vi "Set BG Image.vi"(8 "error in (no error)":errorcluster, 11 "IMAQ Display in":refnum<class "HIJ IMAQdx Display.lvclass">) -> (0 "error out":errorcluster, 3 "IMAQ Display out":refnum<class "HIJ IMAQdx Display.lvclass">)   [LabVIEW 2020, in "HIJ IMAQdx Display.lvlib" / "HIJ IMAQdx Display.lvclass"]
uses:
  HIJ IMAQdx Display.lvclass
  C:/POLARIS Programme/POLARIS-AS-3-Cams/Submodules/HIJ Vision/Display Actors/HIJ Vision Display/HIJ Vision Display/HIJ Vision Display.lvclass
  HIJ IMAQdx Display.lvclass/HIJ IMAQdx Display.ctl
  HIJ Vision Display/HIJ Vision Display/HIJ Vision Display.lvclass/HIJ Vision Display.ctl
  HIJ Vision Display/HIJ Vision Display/Read Image Source Name.vi
  HIJ Vision Display/HIJ Vision Display/Read Display Image.vi
  HIJ Vision Display/HIJ Vision Display/Write Image Name Prefix.vi
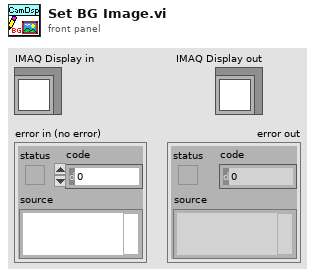
[diagram p1: front panel]
types:
  T1 = typedef "IMAQ Image.ctl" = refnum<image>
  T2 = typedef "Image Type" = u32
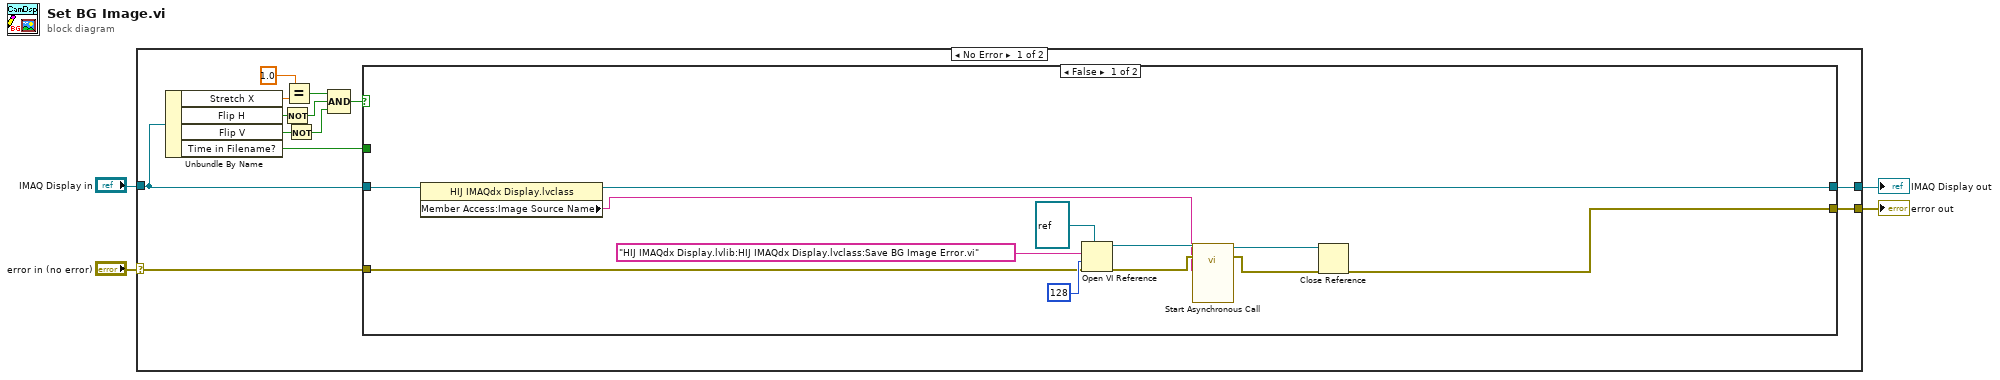
[diagram p0: block diagram]
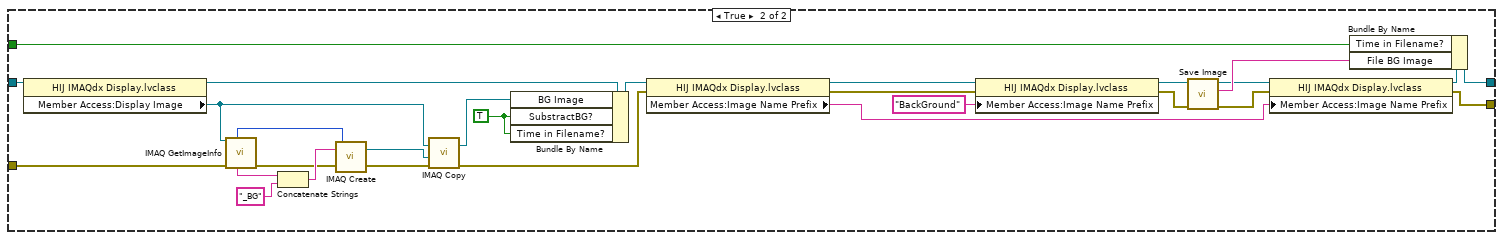
[diagram p2: hidden frame]
diagram:
  n1 = case shown="No Error" "error in (no error)" {
    selector: "error in (no error)" -> [w17 w58]
    tunnel: [w14 w58] -> w3
    tunnel: [w16 w59] -> w1
    tunnel: "IMAQ Display in" -> [w13 w59]
    frame No Error {
      n2 = Unbundle By Name(w13) -> ("Stretch X"=w10:dbl, "Flip H"=w8:bool, "Flip V"=w7:bool, "Time in Filename?"=w15:bool)
      n3 = Not(x=w8) -> (.not. x?=w5:bool)
      n4 = Equal?(x=1.0, y=w10) -> (x = y?=w12:bool)
      n5 = Not(x=w7) -> (.not. x?=w6:bool)
      n6 = Compound Arithmetic op=AND(w12, w5, w6) -> (w9:bool)
      n7 = case shown="False" w9 {
        tunnel: w17 -> [w24 w48]
        tunnel: [w19 w37] -> w16
        tunnel: w15 -> [_ w36]
        tunnel: [w21 w31] -> w14
        tunnel: w13 -> [w29 w30]
        frame False {
          n8 = property class="HIJ IMAQdx Display.lvclass"(reference=w29) -> (reference out=w19:refnum<class "HIJ IMAQdx Display.lvclass">, "Member Access:Image Source Name"=w18:string)  [unwired: 1 in, 1 out]
          n9 = Open VI Reference(type specifier VI Refnum (for type only)=refnum<vi> refnum, vi path="HIJ IMAQdx Display.lvlib:HIJ IMAQdx Display.lvclass:Save BG Image Error.vi" ("String"), options=128, error in (no error)=w24) -> (vi reference=w27:refnum<vi>, error out=w23:errorcluster)  [unwired: 2 in]
          n10 = call-by-ref "Start Asynchronous Call"(reference=w27, error in=w23, "Camera Name"=w18) -> (reference out=w20:refnum<vi>, error out=w22:errorcluster)  [unwired: 11 in]
          n11 = Close Reference(reference=w20, error in (no error)=w22) -> (error out=w21:errorcluster)
        }
        frame True {
          w42 = TRUE ("SubstractBG?")
          n12 = property class="HIJ IMAQdx Display.lvclass"(reference=w30) -> (reference out=w43:refnum<class "HIJ IMAQdx Display.lvclass">, "Member Access:Display Image"=w47:T1)  [unwired: 1 in, 1 out]
          n13 = call "IMAQ GetImageInfo"("error in (no error)"=w48, "Image"=w47) -> ("error out"=w54:errorcluster, "Image Name"=w51:string, "Image Type"=w50:T2)  [unwired: 2 in, 5 out]
          n14 = Concatenate Strings(w51, "_BG" ("string")) -> (w57:string)
          n15 = call "IMAQ Create"("Image Name"=w57, "Image Type"=w50, "error in (no error)"=w54) -> ("New Image"=w53:T1, "error out"=w55:errorcluster)  [unwired: 2 in]
          n16 = call "IMAQ Copy"("error in (no error)"=w55, "Image Dst"=w53, "Image Src"=w47) -> ("error out"=w46:errorcluster, "Image Dst Out"=w49:T1)  [unwired: 3 in]
          n17 = Bundle By Name(cluster=w43, "BG Image"=w49, "SubstractBG?"=w42, "Time in Filename?"=w42) -> (w45:refnum<class "HIJ IMAQdx Display.lvclass">)
          n18 = property class="HIJ IMAQdx Display.lvclass"(reference=w45, error in=w46) -> (reference out=w41:refnum<class "HIJ IMAQdx Display.lvclass">, error out=w38:errorcluster, "Member Access:Image Name Prefix"=w33:string)
          n19 = property class="HIJ IMAQdx Display.lvclass"(reference=w41, error in=w38, "Member Access:Image Name Prefix"="BackGround" ("Image Name Prefix")) -> (reference out=w40:refnum<class "HIJ IMAQdx Display.lvclass">, error out=w35:errorcluster)
          n20 = call-dynamic "Save Image.vi"("error in (no error)"=w35, "IMAQ Display in"=w40) -> ("error out"=w32:errorcluster, "Filename"=w56:string, "IMAQ Display out"=w44:refnum<class "HIJ IMAQdx Display.lvclass">)  [unwired: 7 in]
          n21 = property class="HIJ IMAQdx Display.lvclass"(reference=w44, error in=w32, "Member Access:Image Name Prefix"=w33) -> (reference out=w34:refnum<class "HIJ IMAQdx Display.lvclass">, error out=w31:errorcluster)
          n22 = Bundle By Name(cluster=w34, "Time in Filename?"=w36, "File BG Image"=w56) -> (w37:refnum<class "HIJ IMAQdx Display.lvclass">)
        }
      }
    }
    frame Error {
    }
  }
  "error out" <- w3
  "IMAQ Display out" <- w1
